vi "S4GUI_003.vi"(7 "Tab ObsEng":enum32{"Obs", "CCD modes", "Guider", "Eng"}(tab)) -> ()   [LabVIEW 2018] (continued)
              stop <- TRUE stop-if-true
              n1225 = case shown="False" w351 {
                tunnel: w350 -> [w353 w372]
                tunnel: [w354 w371] -> w347
                tunnel: w349 -> [w356 w370]
                tunnel: [w355 w369] -> w348
                frame True {
                  # "polarimetria"
                  n1226 = case shown="False" w356 {
                    selector: w356 -> [w366 w368]
                    tunnel: [w365 w368] -> w355
                    tunnel: [FALSE FALSE] -> w354
                    tunnel: w353 -> [_ _]
                    frame False {
                      w363 = 11
                      w360 = 80
                      w359 = 12900
                      # "Valor médio\ndo curso do foco."
                      n1227 = local write "Start focus"(w359) -> ()
                      n1228 = local write "Step focus"(w360) -> ()
                      n1229 = local write "#steps"(w363) -> ()
                      n1230 = Quotient & Remainder(x=w363, y=2) -> (floor(x/y)=w361:i32)  [unwired: 1 out]
                      n1231 = Multiply(x=w360, y=w361) -> (x*y=w358:i32)
                      n1232 = Add(x=w359, y=w358) -> (x+y=w357:i32)
                      n1233 = local write "Target focus 2"(w357) -> ()
                      n1234 = local write "Target focus"(w357) -> ()
                      n1235 = Not(x=w366) -> (.not. x?=w365:bool)
                    }
                    frame True {
                    }
                  }
                }
                frame False {
                  # "fotometria"
                  n1236 = case shown="False" w372 {
                    selector: w372 -> [w381 w384]
                    tunnel: [w380 w384] -> w371
                    tunnel: w370 -> [_ _]
                    tunnel: [FALSE FALSE] -> w369
                    frame False {
                      w376 = 11
                      w375 = 100
                      w374 = 13400
                      # "Valor médio\ndo curso do foco."
                      n1237 = local write "Start focus"(w374) -> ()
                      n1238 = local write "Step focus"(w375) -> ()
                      n1239 = local write "#steps"(w376) -> ()
                      n1240 = Quotient & Remainder(x=w376, y=2) -> (floor(x/y)=w378:i32)  [unwired: 1 out]
                      n1241 = Multiply(x=w375, y=w378) -> (x*y=w377:i32)
                      n1242 = Add(x=w374, y=w377) -> (x+y=w373:i32)
                      n1243 = local write "Target focus"(w373) -> ()
                      n1244 = local write "Target focus 2"(w373) -> ()
                      n1245 = Not(x=w381) -> (.not. x?=w380:bool)
                    }
                    frame True {
                    }
                  }
                }
              }
            }
            n1246 = call-dynamic "Read exit.vi"("error in (no error)"=w296, "S4GUI in"=w295) -> ("error out"=w294:errorcluster, "exit"=w293:bool, "S4GUI out"=w292:refnum<class "S4GUI.lvclass">)  [unwired: 7 in]
          }
        }
      }
      event "Lambda Selector": Mouse Down? {
        n1247 = event-data() -> ()  [unwired: 1 in, 7 out]
        n1248 = First Call?() -> (First Call?: T/F=w1992:bool)
        n1249 = case shown="True" w1992 {
          tunnel: w1994 -> [w1996 w1998]
          tunnel: [w1996 w1997] -> w1993
          frame False {
          }
          frame True {
            w2000 = u16 0 items=["OFF", "Lambda/2", "Lambda/4"] ("Lambda Selector")
            n1250 = property on="Lambda Selector" class="Ring (strict)"(error in=w1998, "Value"=w2000) -> (error out=w2001:errorcluster)  [unwired: 1 in, 1 out]
            n1251 = property on="Lambda Selector" class="Ring (strict)"(error in=w2001, "RingText.Text"="OFF" ("Boolean Text.Text")) -> (error out=w1997:errorcluster)  [unwired: 1 in, 1 out]
          }
        }
        n1252 = event-data() -> ()  [unwired: 2 in, 1 out]
      }
      event "object suffix": Key Down; "object suffix": Key Repeat {
        n1253 = event-data() -> ("Char"=w2002:i16)  [unwired: 1 in]
        "charKeyboardInteger" <- w2002
        n1254 = call-dynamic "Write charSuffix.vi"("error in (no error)"=w2005, "charSuffix"=w2002, "S4GUI in"=w2006) -> ("error out"=w2003:errorcluster, "S4GUI out"=w2004:refnum<class "S4GUI.lvclass">)  [unwired: 7 in]
      }
      event "dflat suffix": Key Down; "dflat suffix": Key Repeat {
        n1255 = event-data() -> ("Char"=w2009:i16)  [unwired: 1 in]
        n1256 = call-dynamic "Write charSuffix.vi"("error in (no error)"=w2010, "charSuffix"=w2009, "S4GUI in"=w2011) -> ("error out"=w2007:errorcluster, "S4GUI out"=w2008:refnum<class "S4GUI.lvclass">)  [unwired: 7 in]
      }
      event "sflat suffix": Key Down; "sflat suffix": Key Repeat {
        n1257 = event-data() -> ("Char"=w2014:i16)  [unwired: 1 in]
        n1258 = call-dynamic "Write charSuffix.vi"("error in (no error)"=w2015, "charSuffix"=w2014, "S4GUI in"=w2016) -> ("error out"=w2012:errorcluster, "S4GUI out"=w2013:refnum<class "S4GUI.lvclass">)  [unwired: 7 in]
      }
      event "dark suffix": Key Down; "dark suffix": Key Repeat {
        n1259 = event-data() -> ("Char"=w2019:i16)  [unwired: 1 in]
        n1260 = call-dynamic "Write charSuffix.vi"("error in (no error)"=w2020, "charSuffix"=w2019, "S4GUI in"=w2021) -> ("error out"=w2017:errorcluster, "S4GUI out"=w2018:refnum<class "S4GUI.lvclass">)  [unwired: 7 in]
      }
      event "zero suffix": Key Down; "zero suffix": Key Repeat {
        n1261 = event-data() -> ("Char"=w2024:i16)  [unwired: 1 in]
        n1262 = call-dynamic "Write charSuffix.vi"("error in (no error)"=w2025, "charSuffix"=w2024, "S4GUI in"=w2026) -> ("error out"=w2022:errorcluster, "S4GUI out"=w2023:refnum<class "S4GUI.lvclass">)  [unwired: 7 in]
      }
      event "focus suffix": Key Down; "focus suffix": Key Repeat {
        n1263 = event-data() -> ("Char"=w2029:i16)  [unwired: 1 in]
        n1264 = call-dynamic "Write charSuffix.vi"("error in (no error)"=w2030, "charSuffix"=w2029, "S4GUI in"=w2031) -> ("error out"=w2027:errorcluster, "S4GUI out"=w2028:refnum<class "S4GUI.lvclass">)  [unwired: 7 in]
      }
      event "Set CCD mode": Value Change {
        w2094 = i16 1 items=["Cooler OFF", "Cooler ON"] ("Cooler ON/OFF")
        w2108 = i16 1 items=["Cooler OFF", "Cooler ON"] ("Cooler ON/OFF")
        w2124 = i16 1 items=["Cooler OFF", "Cooler ON"] ("Cooler ON/OFF")
        w2144 = i16 1 items=["Cooler OFF", "Cooler ON"] ("Cooler ON/OFF")
        # "Sinaliza que houve requisição de SET CCD mode"
        n1265 = event-data() -> ()  [unwired: 1 in, 6 out]
        n1266 = call-dynamic "Write User Event.vi"("error in (no error)"=w2302, "User Event"="SET CCD mode ", "S4GUI in"=w2301) -> ("error out"=w2089:errorcluster, "S4GUI out"=w2088:refnum<class "S4GUI.lvclass">)  [unwired: 7 in]
        n1267 = call-dynamic "Write SET request.vi"("error in (no error)"=w2089, "SET request"=TRUE, "S4GUI in"=w2088) -> ("error out"=w2086:errorcluster, "S4GUI out"=w2087:refnum<class "S4GUI.lvclass">)  [unwired: 7 in]
        n1268 = call-dynamic "Read CCD mode.vi"("error in (no error)"=w2086, "S4GUI in"=w2087) -> ("error out"=w2299:errorcluster, "CCD mode"=w2300:T30, "S4GUI out"=w2298:refnum<class "S4GUI.lvclass">)  [unwired: 7 in]
        n1269 = Bundle By Name(cluster=w2300, "FTM"="Frame Transfer", "AQM"="AQM", "SZM"="SZM", "EM gain"="EM Gain") -> (w2297:T30)
        n1270 = call-dynamic "Write CCD mode.vi"("error in (no error)"=w2299, "CCD mode"=w2297, "S4GUI in"=w2298) -> ("error out"=w2155:errorcluster, "S4GUI out"=w2156:refnum<class "S4GUI.lvclass">)  [unwired: 7 in]
        n1271 = call-dynamic "LoadCCDmode.vi"("error in (no error)"=w2155, "S4GUI in"=w2156) -> ("error out"=w2154:errorcluster, "S4GUI out"=w2153:refnum<class "S4GUI.lvclass">)  [unwired: 8 in]
        n1272 = call-dynamic "Read Parameters CCD modes.vi"("error in (no error)"=w2154, "S4GUI in"=w2153) -> ("error out"=w2152:errorcluster, "Parameters CCD modes"=w2157:T5, "S4GUI out"=w2151:refnum<class "S4GUI.lvclass">)  [unwired: 7 in]
        n1273 = Unbundle By Name(w2157) -> ("CCD \nEM Mode"=w2289:u8, "Readout\nRate"=w2149:u8)
        n1274 = case shown="0, Default" w2289 {
          tunnel: [string[] ["30 MHz", "20 MHz", "10 MHz", "1 MHz"] ("Strings []") string[] ["1 MHz", "0.1 MHz"] ("Strings []")] -> w2290
          frame 0, Default {
          }
          frame 1 {
          }
        }
        n1275 = flat-sequence {
          tunnel: w2290 -> [w2436]
          tunnel: w2289 -> [w2437]
          tunnel: [w2437] -> w2291
          tunnel: w2157 -> [w2443]
          tunnel: [w2442] -> w2150
          tunnel: w2291 -> [w2440]
          tunnel: w2158 -> [w2441]
          tunnel: w2149 -> [w2438]
          frame #0 {
            n1276 = property on="Readout\nRate" class="Ring (strict)"("Strings []"=w2436) -> ()  [unwired: 2 in, 2 out]
            n1277 = property on="Readout\nRate" class="Ring (strict)"("Strings []"=w2436) -> ()  [unwired: 2 in, 2 out]
            n1278 = property on="Readout Rate 2" class="Ring (strict)"("Strings []"=w2436) -> ()  [unwired: 2 in, 2 out]
            n1279 = property on="Readout Rate" class="Ring (strict)"("Strings []"=w2436) -> ()  [unwired: 2 in, 2 out]
            n1280 = property on="Readout Rate 3" class="Ring (strict)"("Strings []"=w2436) -> ()  [unwired: 2 in, 2 out]
            n1281 = property on="Readout Rate 4" class="Ring (strict)"("Strings []"=w2436) -> ()  [unwired: 2 in, 2 out]
          }
          frame #1 {
            n1282 = Bundle By Name(cluster=w2443, "Readout\nRate"=w2438, "CCD \nEM Mode"=w2440) -> (w2442:T5)
            n1283 = disable-structure shown="Enabled" {
              disable-tunnel: w2441 -> [w2447 w2448]
              disable-tunnel: w2440 -> [w2446 _]
              disable-tunnel: [w2445 w2448] -> w2439
              disable-tunnel: w2438 -> [w2444 _]
              frame Disabled {
                n1284 = Bundle By Name(cluster=w2447, "Parameters.Readout\nRate"=w2444, "Parameters.CCD \nEM Mode"=w2446) -> (w2445:T8)
              }
              frame Enabled {
              }
            }
            n1285 = local write "Input Cluster"(w2439) -> ()
          }
        }
        n1286 = call-dynamic "Read InfoCCDmode.vi"("error in (no error)"=w2152, "S4GUI in"=w2151) -> ("error out"=w2292:errorcluster, "InfoCCDmode"=w2084:T2, "S4GUI out"=w2293:refnum<class "S4GUI.lvclass">)  [unwired: 7 in]
        "InfoCCDmode" <- w2084
        n1287 = Unbundle By Name(w2084) -> ("MinExpTime"=w2032:dbl)
        n1288 = call-dynamic "Read Parameters CCD modes.vi"("error in (no error)"=w2292, "S4GUI in"=w2293) -> ("error out"=w2286:errorcluster, "Parameters CCD modes"=→"Parameters CCD modes":T5, "S4GUI out"=w2287:refnum<class "S4GUI.lvclass">)  [unwired: 7 in]
        n1289 = local read "Input Cluster"() -> (w2158:T8)
        n1290 = call-dynamic "Write Parameters CCD modes.vi"("error in (no error)"=w2286, "Parameters CCD modes"=w2150, "S4GUI in"=w2287) -> ("error out"=w2265:errorcluster, "S4GUI out"=w2239:refnum<class "S4GUI.lvclass">)  [unwired: 7 in]
        n1291 = Unbundle By Name(w2150) -> ("Frame\nTransfer"=w2193:bool, "Pre-amplification\nGain"=w2192:u8, "Readout\nRate"=w2191:u8, "CCD \nEM Mode"=w2190:u8, "CCD\nEM Gain"=w2189:u16, "Image \nInitial Line"=w2188:u16, "Image\nInitial Column"=w2187:u16, "Image\nFinal Line"=w2176:u16, "Image\nFInal Column"=w2186:u16, "Vertical\nBinning"=w2185:u16, "Horizontal\nBinning"=w2184:u16)
        n1292 = call-dynamic "Read AcquisitionA.vi"("error in (no error)"=w2265, "S4ACS_GUI in"=w2239) -> ("error out"=w2174:errorcluster, "Acquisition.lvclass"=w2175:refnum<class "Acquisition.lvclass">, "S4ACS_GUI out"=w2285:refnum<class "S4GUI.lvclass">)  [unwired: 7 in]
        n1293 = call-dynamic "Read enabled.vi"("error in (no error)"=w2174, "Server in"=w2175) -> ("error out"=w2173:errorcluster, "enabled"=w2171:bool, "Server out"=w2172:refnum<class "Acquisition.lvclass">)  [unwired: 7 in]
        n1294 = call-dynamic "Read Channel.vi"("error in (no error)"=w2173, "Acquisition in"=w2172) -> ("error out"=w2282:errorcluster, "Channel.lvclass"=w2283:refnum<class "Channel.lvclass">, "Acquisition out"=w2284:refnum<class "Acquisition.lvclass">)  [unwired: 7 in]
        n1295 = call-dynamic "Read Interface.vi"("error in (no error)"=w2282, "Channel in"=w2283) -> ("error out"=w2268:errorcluster, "Interface.lvclass"=w2269:refnum<class "Interface.lvclass">, "Channel out"=w2263:refnum<class "Channel.lvclass">)  [unwired: 7 in]
        n1296 = call-dynamic "Write PREV_FT.vi"("error in (no error)"=w2268, "PREV_FT"=w2193, "Interface in"=w2269) -> ("error out"=w2147:errorcluster, "Interface out"=w2146:refnum<class "Interface.lvclass">)  [unwired: 7 in]
        n1297 = call-dynamic "Write Cooler ON_OFF.vi"("error in (no error)"=w2147, "Cooler ON/OFF"=w2144, "Interface in"=w2146) -> ("error out"=w2145:errorcluster, "Interface out"=w2143:refnum<class "Interface.lvclass">)  [unwired: 7 in]
        n1298 = call-dynamic "Read target cluster.vi"("error in (no error)"=w2145, "Channel in"=w2263) -> ("error out"=w2261:errorcluster, "target cluster"=w2260:T31, "Channel out"=w2262:refnum<class "Channel.lvclass">)  [unwired: 7 in]
        n1299 = Bundle By Name(cluster=w2260, "FRAME_TRANSFER"=w2193, "PREAMP"=w2192, "READOUT_RATE"=w2191, "EM_MODE"=w2190, "EM_GAIN"=w2189, "INITIAL_LINE"=w2188, "INITIAL_COLUMN"=w2187, "FINAL_LINE"=w2176, "FINAL_COLUMN"=w2186, "VBIN"=w2185, "HBIN"=w2184) -> (w2140:T31)
        n1300 = call-dynamic "Write target cluster.vi"("error in (no error)"=w2261, "target cluster"=w2140, "Channel in"=w2262) -> ("error out"=w2141:errorcluster, "Channel out"=w2267:refnum<class "Channel.lvclass">)  [unwired: 7 in]
        n1301 = call-dynamic "Set CCD_Config.vi"("error in (no error)"=w2141, "input cluster"=w2140, "Interface in"=w2143) -> ("error out"=w2130:errorcluster, "Interface out"=w2142:refnum<class "Interface.lvclass">)  [unwired: 7 in]
        n1302 = Flatten To String(anything=w2140, error in (no error)=w2141) -> (data string=w2277:string)  [unwired: 2 in, 2 out]
        n1303 = call "Write flatted cluster.vi"("error in (no error)"=w2130, "flatted cluster"=w2277, "Interface in"=w2142) -> ("error out"=w2079:errorcluster, "Interface out"=w2080:refnum<class "Interface.lvclass">)  [unwired: 7 in]
        n1304 = call "Read Exposure Time.vi"("error in (no error)"=w2079, "Interface in"=w2080) -> ("error out"=w2077:errorcluster, "Exposure Time"=w2082:dbl, "Interface out"=w2078:refnum<class "Interface.lvclass">)  [unwired: 7 in]
        n1305 = Greater Or Equal?(x=w2082, y=w2032) -> (x >= y?=w2083:bool)
        n1306 = Select(t=w2082, s=w2083, f=w2032) -> (s? t:f=w2081:dbl)
        n1307 = local write "Exptime ch1"(w2081) -> ()
        n1308 = call "Write Exposure Time.vi"("error in (no error)"=w2077, "Exposure Time"=w2081, "Interface in"=w2078) -> ("error out"=w2076:errorcluster, "Interface out"=w2075:refnum<class "Interface.lvclass">)  [unwired: 7 in]
        n1309 = call-dynamic "Write Interface.vi"("error in (no error)"=w2076, "Interface.lvclass"=w2075, "Channel in"=w2267) -> ("error out"=w2273:errorcluster, "Channel out"=w2275:refnum<class "Channel.lvclass">)  [unwired: 7 in]
        n1310 = call "Write section_name.vi"("error in (no error)"=w2273, "section_name"="CCD_ACS1", "Channel in"=w2275) -> ("error out"=w2272:errorcluster, "Channel out"=w2274:refnum<class "Channel.lvclass">)  [unwired: 7 in]
        n1311 = call-dynamic "save config.vi"("error in (no error)"=w2272, "file config"="lastsaved.cfg", "Channel in"=w2274) -> ("error out"=w2138:errorcluster, "Channel out"=w2139:refnum<class "Channel.lvclass">)  [unwired: 7 in]
        n1312 = call-dynamic "ValidateConfig.vi"("error in (no error)"=w2138, "Channel in"=w2139) -> ("error out"=w2136:errorcluster, "Channel out"=w2137:refnum<class "Channel.lvclass">)  [unwired: 7 in, 1 out]
        n1313 = call-dynamic "Save Temp.vi"("error in (no error)"=w2136, "temp file"="lasttemp.cfg" ("file config"), "Channel in"=w2137) -> ("error out"=w2135:errorcluster, "Channel out"=w2134:refnum<class "Channel.lvclass">)  [unwired: 7 in]
        n1314 = case shown="True" w2171 {
          tunnel: [w2404 w2429] -> w2281
          tunnel: [w2403 w2428] -> w2280
          tunnel: w2134 -> [w2404 w2427]
          tunnel: w2135 -> [w2403 w2426]
          frame False {
          }
          frame True {
            # "Esvazia\na fila."
            n1315 = call-dynamic "Read State Machine.vi"("error in (no error)"=w2426, "Device in"=w2427) -> ("error out"=w2420:errorcluster, "State Machine.lvclass"=w2423:refnum<class "State Machine.lvclass">, "Device out"=w2433:refnum<class "Channel.lvclass">)  [unwired: 7 in]
            n1316 = call-dynamic "Read ref StatesQueue.vi"("error in (no error)"=w2420, "State Machine in"=w2423) -> ("error out"=w2411:errorcluster, "ref StatesQueue"=w2413:refnum<queue>, "State Machine out"=w2422:refnum<class "State Machine.lvclass">)  [unwired: 7 in]
            n1317 = Flush Queue(queue=w2413, error in (no error)=w2411) -> (queue out=w2412:refnum<queue>, error out=w2410:errorcluster)  [unwired: 1 out]
            n1318 = Enqueue Element(queue=w2412, element=u32 60 ("State"), error in (no error)=w2410) -> (queue out=w2425:refnum<queue>, error out=w2419:errorcluster)  [unwired: 1 in, 1 out]
            n1319 = Enqueue Element(queue=w2425, element=u32 45 ("State"), error in (no error)=w2419) -> (queue out=w2424:refnum<queue>, error out=w2418:errorcluster)  [unwired: 1 in, 1 out]
            n1320 = Enqueue Element(queue=w2424, element=u32 35 ("State"), error in (no error)=w2418) -> (queue out=w2408:refnum<queue>, error out=w2407:errorcluster)  [unwired: 1 in, 1 out]
            n1321 = Enqueue Element(queue=w2408, element=u32 37 ("State"), error in (no error)=w2407) -> (queue out=w2405:refnum<queue>, error out=w2406:errorcluster)  [unwired: 1 in, 1 out]
            n1322 = call-dynamic "Write ref StatesQueue.vi"("error in (no error)"=w2406, "ref StatesQueue"=w2405, "State Machine in"=w2422) -> ("error out"=w2414:errorcluster, "State Machine out"=w2421:refnum<class "State Machine.lvclass">)  [unwired: 7 in]
            n1323 = disable-structure shown="Enabled" {
              disable-tunnel: [0 ("State") 45] -> w2430
              frame Enabled {
                # "Vai pra 0 para que\nos estados da fila \nsejam retirados."
              }
              frame Disabled {
                # "Verifica Texp\nantes de tudo."
              }
            }
            n1324 = call-dynamic "Write State.vi"("error in (no error)"=w2414, "State"=w2430, "State Machine in"=w2421) -> ("error out"=w2431:errorcluster, "State Machine out"=w2432:refnum<class "State Machine.lvclass">)  [unwired: 7 in]
            n1325 = call-dynamic "Write State Machine.vi"("error in (no error)"=w2431, "State Machine.lvclass"=w2432, "Device in"=w2433) -> ("error out"=w2428:errorcluster, "Device out"=w2429:refnum<class "Channel.lvclass">)  [unwired: 7 in]
          }
        }
        n1326 = call-dynamic "Write Channel.vi"("error in (no error)"=w2280, "Channel.lvclass"=w2281, "Acquisition in"=w2284) -> ("error out"=w2279:errorcluster, "Acquisition out"=w2278:refnum<class "Acquisition.lvclass">)  [unwired: 7 in]
        n1327 = call-dynamic "Write AcquisitionA.vi"("error in (no error)"=w2279, "Acquisition.lvclass"=w2278, "S4ACS_GUI in"=w2285) -> ("error out"=w2181:errorcluster, "S4ACS_GUI out"=w2238:refnum<class "S4GUI.lvclass">)  [unwired: 7 in]
        n1328 = call "Read AcquisitionB.vi"("error in (no error)"=errorcluster {"status"=FALSE, "code"=0, "source"=""}, "S4ACS_GUI in"=w2238) -> ("error out"=w2167:errorcluster, "Acquisition.lvclass"=w2170:refnum<class "Acquisition.lvclass">, "S4ACS_GUI out"=w2259:refnum<class "S4GUI.lvclass">)  [unwired: 7 in]
        n1329 = call-dynamic "Read enabled.vi"("error in (no error)"=w2167, "Server in"=w2170) -> ("error out"=w2168:errorcluster, "enabled"=w2060:bool, "Server out"=w2169:refnum<class "Acquisition.lvclass">)  [unwired: 7 in]
        n1330 = call-dynamic "Read Channel.vi"("error in (no error)"=w2168, "Acquisition in"=w2169) -> ("error out"=w2256:errorcluster, "Channel.lvclass"=w2257:refnum<class "Channel.lvclass">, "Acquisition out"=w2258:refnum<class "Acquisition.lvclass">)  [unwired: 7 in]
        n1331 = call-dynamic "Read Interface.vi"("error in (no error)"=w2256, "Channel in"=w2257) -> ("error out"=w2245:errorcluster, "Interface.lvclass"=w2246:refnum<class "Interface.lvclass">, "Channel out"=w2243:refnum<class "Channel.lvclass">)  [unwired: 7 in]
        n1332 = call-dynamic "Write PREV_FT.vi"("error in (no error)"=w2245, "PREV_FT"=w2193, "Interface in"=w2246) -> ("error out"=w2125:errorcluster, "Interface out"=w2127:refnum<class "Interface.lvclass">)  [unwired: 7 in]
        n1333 = call-dynamic "Write Cooler ON_OFF.vi"("error in (no error)"=w2125, "Cooler ON/OFF"=w2124, "Interface in"=w2127) -> ("error out"=w2123:errorcluster, "Interface out"=w2126:refnum<class "Interface.lvclass">)  [unwired: 7 in]
        n1334 = call-dynamic "Read target cluster.vi"("error in (no error)"=w2123, "Channel in"=w2243) -> ("error out"=w2241:errorcluster, "target cluster"=w2240:T31, "Channel out"=w2242:refnum<class "Channel.lvclass">)  [unwired: 7 in]
        n1335 = Bundle By Name(cluster=w2240, "FRAME_TRANSFER"=w2193, "PREAMP"=w2192, "READOUT_RATE"=w2191, "EM_MODE"=w2190, "EM_GAIN"=w2189, "INITIAL_LINE"=w2188, "INITIAL_COLUMN"=w2187, "FINAL_LINE"=w2176, "FINAL_COLUMN"=w2186, "VBIN"=w2185, "HBIN"=w2184) -> (w2128:T31)
        n1336 = call-dynamic "Write target cluster.vi"("error in (no error)"=w2241, "target cluster"=w2128, "Channel in"=w2242) -> ("error out"=w2131:errorcluster, "Channel out"=w2244:refnum<class "Channel.lvclass">)  [unwired: 7 in]
        n1337 = call-dynamic "Set CCD_Config.vi"("error in (no error)"=w2131, "input cluster"=w2128, "Interface in"=w2126) -> ("error out"=w2129:errorcluster, "Interface out"=w2132:refnum<class "Interface.lvclass">)  [unwired: 7 in]
        n1338 = Flatten To String(anything=w2128, error in (no error)=w2131) -> (data string=w2253:string)  [unwired: 2 in, 2 out]
        n1339 = call "Write flatted cluster.vi"("error in (no error)"=w2129, "flatted cluster"=w2253, "Interface in"=w2132) -> ("error out"=w2053:errorcluster, "Interface out"=w2054:refnum<class "Interface.lvclass">)  [unwired: 7 in]
        n1340 = call "Read Exposure Time.vi"("error in (no error)"=w2053, "Interface in"=w2054) -> ("error out"=w2074:errorcluster, "Exposure Time"=w2055:dbl, "Interface out"=w2073:refnum<class "Interface.lvclass">)  [unwired: 7 in]
        n1341 = Greater Or Equal?(x=w2055, y=w2032) -> (x >= y?=w2071:bool)
        n1342 = Select(t=w2055, s=w2071, f=w2032) -> (s? t:f=w2072:dbl)
        n1343 = local write "Exptime ch2"(w2072) -> ()
        n1344 = call "Write Exposure Time.vi"("error in (no error)"=w2074, "Exposure Time"=w2072, "Interface in"=w2073) -> ("error out"=w2052:errorcluster, "Interface out"=w2051:refnum<class "Interface.lvclass">)  [unwired: 7 in]
        n1345 = call-dynamic "Write Interface.vi"("error in (no error)"=w2052, "Interface.lvclass"=w2051, "Channel in"=w2244) -> ("error out"=w2249:errorcluster, "Channel out"=w2251:refnum<class "Channel.lvclass">)  [unwired: 7 in]
        n1346 = call "Write section_name.vi"("error in (no error)"=w2249, "section_name"="CCD_ACS2", "Channel in"=w2251) -> ("error out"=w2248:errorcluster, "Channel out"=w2250:refnum<class "Channel.lvclass">)  [unwired: 7 in]
        n1347 = call-dynamic "save config.vi"("error in (no error)"=w2248, "file config"="lastsaved.cfg", "Channel in"=w2250) -> ("error out"=w2118:errorcluster, "Channel out"=w2119:refnum<class "Channel.lvclass">)  [unwired: 7 in]
        n1348 = call-dynamic "ValidateConfig.vi"("error in (no error)"=w2118, "Channel in"=w2119) -> ("error out"=w2121:errorcluster, "Channel out"=w2122:refnum<class "Channel.lvclass">)  [unwired: 7 in, 1 out]
        n1349 = call-dynamic "Save Temp.vi"("error in (no error)"=w2121, "temp file"="lasttemp.cfg" ("file config"), "Channel in"=w2122) -> ("error out"=w2058:errorcluster, "Channel out"=w2059:refnum<class "Channel.lvclass">)  [unwired: 7 in]
        n1350 = case shown="True" w2060 {
          tunnel: [w2338 w2363] -> w2057
          tunnel: [w2337 w2362] -> w2056
          tunnel: w2059 -> [w2338 w2361]
          tunnel: w2058 -> [w2337 w2360]
          frame False {
          }
          frame True {
            # "Esvazia\na fila."
            n1351 = call-dynamic "Read State Machine.vi"("error in (no error)"=w2360, "Device in"=w2361) -> ("error out"=w2354:errorcluster, "State Machine.lvclass"=w2357:refnum<class "State Machine.lvclass">, "Device out"=w2367:refnum<class "Channel.lvclass">)  [unwired: 7 in]
            n1352 = call-dynamic "Read ref StatesQueue.vi"("error in (no error)"=w2354, "State Machine in"=w2357) -> ("error out"=w2344:errorcluster, "ref StatesQueue"=w2346:refnum<queue>, "State Machine out"=w2356:refnum<class "State Machine.lvclass">)  [unwired: 7 in]
            n1353 = Flush Queue(queue=w2346, error in (no error)=w2344) -> (queue out=w2345:refnum<queue>, error out=w2343:errorcluster)  [unwired: 1 out]
            n1354 = Enqueue Element(queue=w2345, element=u32 60 ("State"), error in (no error)=w2343) -> (queue out=w2359:refnum<queue>, error out=w2353:errorcluster)  [unwired: 1 in, 1 out]
            n1355 = Enqueue Element(queue=w2359, element=u32 45 ("State"), error in (no error)=w2353) -> (queue out=w2358:refnum<queue>, error out=w2352:errorcluster)  [unwired: 1 in, 1 out]
            n1356 = Enqueue Element(queue=w2358, element=u32 35 ("State"), error in (no error)=w2352) -> (queue out=w2351:refnum<queue>, error out=w2341:errorcluster)  [unwired: 1 in, 1 out]
            n1357 = Enqueue Element(queue=w2351, element=u32 37, error in (no error)=w2341) -> (queue out=w2342:refnum<queue>, error out=w2340:errorcluster)  [unwired: 1 in, 1 out]
            n1358 = call-dynamic "Write ref StatesQueue.vi"("error in (no error)"=w2340, "ref StatesQueue"=w2342, "State Machine in"=w2356) -> ("error out"=w2347:errorcluster, "State Machine out"=w2355:refnum<class "State Machine.lvclass">)  [unwired: 7 in]
            n1359 = disable-structure shown="Enabled" {
              disable-tunnel: [0 ("State") 45] -> w2364
              frame Enabled {
                # "Vai pra 0 para que\nos estados da fila \nsejam retirados."
              }
              frame Disabled {
                # "Verifica Texp\nantes de tudo."
              }
            }
            n1360 = call-dynamic "Write State.vi"("error in (no error)"=w2347, "State"=w2364, "State Machine in"=w2355) -> ("error out"=w2365:errorcluster, "State Machine out"=w2366:refnum<class "State Machine.lvclass">)  [unwired: 7 in]
            n1361 = call-dynamic "Write State Machine.vi"("error in (no error)"=w2365, "State Machine.lvclass"=w2366, "Device in"=w2367) -> ("error out"=w2362:errorcluster, "Device out"=w2363:refnum<class "Channel.lvclass">)  [unwired: 7 in]
          }
        }
        n1362 = call-dynamic "Write Channel.vi"("error in (no error)"=w2056, "Channel.lvclass"=w2057, "Acquisition in"=w2258) -> ("error out"=w2255:errorcluster, "Acquisition out"=w2254:refnum<class "Acquisition.lvclass">)  [unwired: 7 in]
        n1363 = call "Write AcquisitionB.vi"("error in (no error)"=w2255, "Acquisition.lvclass"=w2254, "S4ACS_GUI in"=w2259) -> ("error out"=w2180:errorcluster, "S4ACS_GUI out"=w2215:refnum<class "S4GUI.lvclass">)  [unwired: 7 in]
        n1364 = call-dynamic "Read AcquisitionC.vi"("error in (no error)"=errorcluster {"status"=FALSE, "code"=0, "source"=""}, "S4ACS_GUI in"=w2215) -> ("error out"=w2164:errorcluster, "Acquisition.lvclass"=w2166:refnum<class "Acquisition.lvclass">, "S4ACS_GUI out"=w2236:refnum<class "S4GUI.lvclass">)  [unwired: 7 in]
        n1365 = call-dynamic "Read enabled.vi"("error in (no error)"=w2164, "Server in"=w2166) -> ("error out"=w2163:errorcluster, "enabled"=w2050:bool, "Server out"=w2165:refnum<class "Acquisition.lvclass">)  [unwired: 7 in]
        n1366 = call-dynamic "Read Channel.vi"("error in (no error)"=w2163, "Acquisition in"=w2165) -> ("error out"=w2233:errorcluster, "Channel.lvclass"=w2234:refnum<class "Channel.lvclass">, "Acquisition out"=w2235:refnum<class "Acquisition.lvclass">)  [unwired: 7 in]
        n1367 = call-dynamic "Read Interface.vi"("error in (no error)"=w2233, "Channel in"=w2234) -> ("error out"=w2222:errorcluster, "Interface.lvclass"=w2223:refnum<class "Interface.lvclass">, "Channel out"=w2220:refnum<class "Channel.lvclass">)  [unwired: 7 in]
        n1368 = call-dynamic "Write PREV_FT.vi"("error in (no error)"=w2222, "PREV_FT"=w2193, "Interface in"=w2223) -> ("error out"=w2105:errorcluster, "Interface out"=w2107:refnum<class "Interface.lvclass">)  [unwired: 7 in]
        n1369 = call-dynamic "Write Cooler ON_OFF.vi"("error in (no error)"=w2105, "Cooler ON/OFF"=w2108, "Interface in"=w2107) -> ("error out"=w2104:errorcluster, "Interface out"=w2106:refnum<class "Interface.lvclass">)  [unwired: 7 in]
        n1370 = call-dynamic "Read target cluster.vi"("error in (no error)"=w2104, "Channel in"=w2220) -> ("error out"=w2218:errorcluster, "target cluster"=w2217:T31, "Channel out"=w2219:refnum<class "Channel.lvclass">)  [unwired: 7 in]
        n1371 = Bundle By Name(cluster=w2217, "FRAME_TRANSFER"=w2193, "PREAMP"=w2192, "READOUT_RATE"=w2191, "EM_MODE"=w2190, "EM_GAIN"=w2189, "INITIAL_LINE"=w2188, "INITIAL_COLUMN"=w2187, "FINAL_LINE"=w2176, "FINAL_COLUMN"=w2186, "VBIN"=w2185, "HBIN"=w2184) -> (w2112:T31)
        n1372 = call-dynamic "Write target cluster.vi"("error in (no error)"=w2218, "target cluster"=w2112, "Channel in"=w2219) -> ("error out"=w2111:errorcluster, "Channel out"=w2221:refnum<class "Channel.lvclass">)  [unwired: 7 in]
        n1373 = call-dynamic "Set CCD_Config.vi"("error in (no error)"=w2111, "input cluster"=w2112, "Interface in"=w2106) -> ("error out"=w2110:errorcluster, "Interface out"=w2109:refnum<class "Interface.lvclass">)  [unwired: 7 in]
        n1374 = Flatten To String(anything=w2112, error in (no error)=w2111) -> (data string=w2230:string)  [unwired: 2 in, 2 out]
        n1375 = call "Write flatted cluster.vi"("error in (no error)"=w2110, "flatted cluster"=w2230, "Interface in"=w2109) -> ("error out"=w2044:errorcluster, "Interface out"=w2045:refnum<class "Interface.lvclass">)  [unwired: 7 in]
        n1376 = call "Read Exposure Time.vi"("error in (no error)"=w2044, "Interface in"=w2045) -> ("error out"=w2066:errorcluster, "Exposure Time"=w2069:dbl, "Interface out"=w2067:refnum<class "Interface.lvclass">)  [unwired: 7 in]
        n1377 = Greater Or Equal?(x=w2069, y=w2032) -> (x >= y?=w2070:bool)
        n1378 = Select(t=w2069, s=w2070, f=w2032) -> (s? t:f=w2068:dbl)
        n1379 = local write "Exptime ch3"(w2068) -> ()
        n1380 = call "Write Exposure Time.vi"("error in (no error)"=w2066, "Exposure Time"=w2068, "Interface in"=w2067) -> ("error out"=w2042:errorcluster, "Interface out"=w2043:refnum<class "Interface.lvclass">)  [unwired: 7 in]
        n1381 = call-dynamic "Write Interface.vi"("error in (no error)"=w2042, "Interface.lvclass"=w2043, "Channel in"=w2221) -> ("error out"=w2226:errorcluster, "Channel out"=w2228:refnum<class "Channel.lvclass">)  [unwired: 7 in]
        n1382 = call "Write section_name.vi"("error in (no error)"=w2226, "section_name"="CCD_ACS3", "Channel in"=w2228) -> ("error out"=w2225:errorcluster, "Channel out"=w2227:refnum<class "Channel.lvclass">)  [unwired: 7 in]
        n1383 = call-dynamic "save config.vi"("error in (no error)"=w2225, "file config"="lastsaved.cfg", "Channel in"=w2227) -> ("error out"=w2113:errorcluster, "Channel out"=w2114:refnum<class "Channel.lvclass">)  [unwired: 7 in]
        n1384 = call-dynamic "ValidateConfig.vi"("error in (no error)"=w2113, "Channel in"=w2114) -> ("error out"=w2116:errorcluster, "Channel out"=w2117:refnum<class "Channel.lvclass">)  [unwired: 7 in, 1 out]
        n1385 = call-dynamic "Save Temp.vi"("error in (no error)"=w2116, "temp file"="lasttemp.cfg" ("file config"), "Channel in"=w2117) -> ("error out"=w2048:errorcluster, "Channel out"=w2049:refnum<class "Channel.lvclass">)  [unwired: 7 in]
        n1386 = case shown="True" w2050 {
          tunnel: [w2305 w2330] -> w2047
          tunnel: [w2304 w2329] -> w2046
          tunnel: w2049 -> [w2305 w2328]
          tunnel: w2048 -> [w2304 w2327]
          frame False {
          }
          frame True {
            # "Esvazia\na fila."
            n1387 = call-dynamic "Read State Machine.vi"("error in (no error)"=w2327, "Device in"=w2328) -> ("error out"=w2321:errorcluster, "State Machine.lvclass"=w2324:refnum<class "State Machine.lvclass">, "Device out"=w2334:refnum<class "Channel.lvclass">)  [unwired: 7 in]
            n1388 = call-dynamic "Read ref StatesQueue.vi"("error in (no error)"=w2321, "State Machine in"=w2324) -> ("error out"=w2311:errorcluster, "ref StatesQueue"=w2313:refnum<queue>, "State Machine out"=w2323:refnum<class "State Machine.lvclass">)  [unwired: 7 in]
            n1389 = Flush Queue(queue=w2313, error in (no error)=w2311) -> (queue out=w2312:refnum<queue>, error out=w2310:errorcluster)  [unwired: 1 out]
            n1390 = Enqueue Element(queue=w2312, element=u32 60 ("State"), error in (no error)=w2310) -> (queue out=w2326:refnum<queue>, error out=w2320:errorcluster)  [unwired: 1 in, 1 out]
            n1391 = Enqueue Element(queue=w2326, element=u32 45 ("State"), error in (no error)=w2320) -> (queue out=w2325:refnum<queue>, error out=w2319:errorcluster)  [unwired: 1 in, 1 out]
            n1392 = Enqueue Element(queue=w2325, element=u32 35 ("State"), error in (no error)=w2319) -> (queue out=w2318:refnum<queue>, error out=w2308:errorcluster)  [unwired: 1 in, 1 out]
            n1393 = Enqueue Element(queue=w2318, element=u32 37, error in (no error)=w2308) -> (queue out=w2309:refnum<queue>, error out=w2307:errorcluster)  [unwired: 1 in, 1 out]
            n1394 = call-dynamic "Write ref StatesQueue.vi"("error in (no error)"=w2307, "ref StatesQueue"=w2309, "State Machine in"=w2323) -> ("error out"=w2314:errorcluster, "State Machine out"=w2322:refnum<class "State Machine.lvclass">)  [unwired: 7 in]
            n1395 = disable-structure shown="Enabled" {
              disable-tunnel: [0 ("State") 45] -> w2331
              frame Enabled {
                # "Vai pra 0 para que\nos estados da fila \nsejam retirados."
              }
              frame Disabled {
                # "Verifica Texp\nantes de tudo."
              }
            }
            n1396 = call-dynamic "Write State.vi"("error in (no error)"=w2314, "State"=w2331, "State Machine in"=w2322) -> ("error out"=w2332:errorcluster, "State Machine out"=w2333:refnum<class "State Machine.lvclass">)  [unwired: 7 in]
            n1397 = call-dynamic "Write State Machine.vi"("error in (no error)"=w2332, "State Machine.lvclass"=w2333, "Device in"=w2334) -> ("error out"=w2329:errorcluster, "Device out"=w2330:refnum<class "Channel.lvclass">)  [unwired: 7 in]
          }
        }
        n1398 = call-dynamic "Write Channel.vi"("error in (no error)"=w2046, "Channel.lvclass"=w2047, "Acquisition in"=w2235) -> ("error out"=w2232:errorcluster, "Acquisition out"=w2231:refnum<class "Acquisition.lvclass">)  [unwired: 7 in]
        n1399 = call-dynamic "Write AcquisitionC.vi"("error in (no error)"=w2232, "Acquisition.lvclass"=w2231, "S4ACS_GUI in"=w2236) -> ("error out"=w2179:errorcluster, "S4ACS_GUI out"=w2183:refnum<class "S4GUI.lvclass">)  [unwired: 7 in]
        n1400 = call-dynamic "Read AcquisitionD.vi"("error in (no error)"=errorcluster {"status"=FALSE, "code"=0, "source"=""}, "S4ACS_GUI in"=w2183) -> ("error out"=w2160:errorcluster, "Acquisition.lvclass"=w2162:refnum<class "Acquisition.lvclass">, "S4ACS_GUI out"=w2214:refnum<class "S4GUI.lvclass">)  [unwired: 7 in]
        n1401 = call-dynamic "Read enabled.vi"("error in (no error)"=w2160, "Server in"=w2162) -> ("error out"=w2159:errorcluster, "enabled"=w2041:bool, "Server out"=w2161:refnum<class "Acquisition.lvclass">)  [unwired: 7 in]
        n1402 = call-dynamic "Read Channel.vi"("error in (no error)"=w2159, "Acquisition in"=w2161) -> ("error out"=w2211:errorcluster, "Channel.lvclass"=w2212:refnum<class "Channel.lvclass">, "Acquisition out"=w2213:refnum<class "Acquisition.lvclass">)  [unwired: 7 in]
        n1403 = call-dynamic "Read Interface.vi"("error in (no error)"=w2211, "Channel in"=w2212) -> ("error out"=w2200:errorcluster, "Interface.lvclass"=w2201:refnum<class "Interface.lvclass">, "Channel out"=w2198:refnum<class "Channel.lvclass">)  [unwired: 7 in]
        n1404 = call-dynamic "Write PREV_FT.vi"("error in (no error)"=w2200, "PREV_FT"=w2193, "Interface in"=w2201) -> ("error out"=w2093:errorcluster, "Interface out"=w2092:refnum<class "Interface.lvclass">)  [unwired: 7 in]
        n1405 = call-dynamic "Write Cooler ON_OFF.vi"("error in (no error)"=w2093, "Cooler ON/OFF"=w2094, "Interface in"=w2092) -> ("error out"=w2090:errorcluster, "Interface out"=w2091:refnum<class "Interface.lvclass">)  [unwired: 7 in]
        n1406 = call-dynamic "Read target cluster.vi"("error in (no error)"=w2090, "Channel in"=w2198) -> ("error out"=w2196:errorcluster, "target cluster"=w2195:T31, "Channel out"=w2197:refnum<class "Channel.lvclass">)  [unwired: 7 in]
        n1407 = Bundle By Name(cluster=w2195, "FRAME_TRANSFER"=w2193, "PREAMP"=w2192, "READOUT_RATE"=w2191, "EM_MODE"=w2190, "EM_GAIN"=w2189, "INITIAL_LINE"=w2188, "INITIAL_COLUMN"=w2187, "FINAL_LINE"=w2176, "FINAL_COLUMN"=w2186, "VBIN"=w2185, "HBIN"=w2184) -> (w2095:T31)
        n1408 = call-dynamic "Write target cluster.vi"("error in (no error)"=w2196, "target cluster"=w2095, "Channel in"=w2197) -> ("error out"=w2096:errorcluster, "Channel out"=w2199:refnum<class "Channel.lvclass">)  [unwired: 7 in]
        n1409 = call-dynamic "Set CCD_Config.vi"("error in (no error)"=w2096, "input cluster"=w2095, "Interface in"=w2091) -> ("error out"=w2097:errorcluster, "Interface out"=w2098:refnum<class "Interface.lvclass">)  [unwired: 7 in]
        n1410 = Flatten To String(anything=w2095, error in (no error)=w2096) -> (data string=w2208:string)  [unwired: 2 in, 2 out]
        n1411 = call "Write flatted cluster.vi"("error in (no error)"=w2097, "flatted cluster"=w2208, "Interface in"=w2098) -> ("error out"=w2035:errorcluster, "Interface out"=w2036:refnum<class "Interface.lvclass">)  [unwired: 7 in]
        n1412 = call "Read Exposure Time.vi"("error in (no error)"=w2035, "Interface in"=w2036) -> ("error out"=w2065:errorcluster, "Exposure Time"=w2062:dbl, "Interface out"=w2064:refnum<class "Interface.lvclass">)  [unwired: 7 in]
        n1413 = Greater Or Equal?(x=w2062, y=w2032) -> (x >= y?=w2061:bool)
        n1414 = Select(t=w2062, s=w2061, f=w2032) -> (s? t:f=w2063:dbl)
        n1415 = local write "Exptime ch4"(w2063) -> ()
        n1416 = call "Write Exposure Time.vi"("error in (no error)"=w2065, "Exposure Time"=w2063, "Interface in"=w2064) -> ("error out"=w2033:errorcluster, "Interface out"=w2034:refnum<class "Interface.lvclass">)  [unwired: 7 in]
        n1417 = call-dynamic "Write Interface.vi"("error in (no error)"=w2033, "Interface.lvclass"=w2034, "Channel in"=w2199) -> ("error out"=w2204:errorcluster, "Channel out"=w2206:refnum<class "Channel.lvclass">)  [unwired: 7 in]
        n1418 = call "Write section_name.vi"("error in (no error)"=w2204, "section_name"="CCD_ACS4", "Channel in"=w2206) -> ("error out"=w2203:errorcluster, "Channel out"=w2205:refnum<class "Channel.lvclass">)  [unwired: 7 in]
        n1419 = call-dynamic "save config.vi"("error in (no error)"=w2203, "file config"="lastsaved.cfg", "Channel in"=w2205) -> ("error out"=w2099:errorcluster, "Channel out"=w2100:refnum<class "Channel.lvclass">)  [unwired: 7 in]
        n1420 = call-dynamic "ValidateConfig.vi"("error in (no error)"=w2099, "Channel in"=w2100) -> ("error out"=w2102:errorcluster, "Channel out"=w2103:refnum<class "Channel.lvclass">)  [unwired: 7 in, 1 out]
        n1421 = call-dynamic "Save Temp.vi"("error in (no error)"=w2102, "temp file"="lasttemp.cfg" ("file config"), "Channel in"=w2103) -> ("error out"=w2038:errorcluster, "Channel out"=w2037:refnum<class "Channel.lvclass">)  [unwired: 7 in]
        n1422 = case shown="True" w2041 {
          tunnel: [w2370 w2396] -> w2040
          tunnel: [w2371 w2395] -> w2039
          tunnel: w2038 -> [w2371 w2394]
          tunnel: w2037 -> [w2370 w2376]
          frame False {
          }
          frame True {
            # "Esvazia\na fila."
            n1423 = call-dynamic "Read State Machine.vi"("error in (no error)"=w2394, "Device in"=w2376) -> ("error out"=w2388:errorcluster, "State Machine.lvclass"=w2391:refnum<class "State Machine.lvclass">, "Device out"=w2400:refnum<class "Channel.lvclass">)  [unwired: 7 in]
            n1424 = call-dynamic "Read ref StatesQueue.vi"("error in (no error)"=w2388, "State Machine in"=w2391) -> ("error out"=w2378:errorcluster, "ref StatesQueue"=w2380:refnum<queue>, "State Machine out"=w2390:refnum<class "State Machine.lvclass">)  [unwired: 7 in]
            n1425 = Flush Queue(queue=w2380, error in (no error)=w2378) -> (queue out=w2379:refnum<queue>, error out=w2377:errorcluster)  [unwired: 1 out]
            n1426 = Enqueue Element(queue=w2379, element=u32 60 ("State"), error in (no error)=w2377) -> (queue out=w2393:refnum<queue>, error out=w2387:errorcluster)  [unwired: 1 in, 1 out]
            n1427 = Enqueue Element(queue=w2393, element=u32 45 ("State"), error in (no error)=w2387) -> (queue out=w2392:refnum<queue>, error out=w2386:errorcluster)  [unwired: 1 in, 1 out]
            n1428 = Enqueue Element(queue=w2392, element=u32 35 ("State"), error in (no error)=w2386) -> (queue out=w2385:refnum<queue>, error out=w2374:errorcluster)  [unwired: 1 in, 1 out]
            n1429 = Enqueue Element(queue=w2385, element=u32 37, error in (no error)=w2374) -> (queue out=w2375:refnum<queue>, error out=w2373:errorcluster)  [unwired: 1 in, 1 out]
            n1430 = call-dynamic "Write ref StatesQueue.vi"("error in (no error)"=w2373, "ref StatesQueue"=w2375, "State Machine in"=w2390) -> ("error out"=w2381:errorcluster, "State Machine out"=w2389:refnum<class "State Machine.lvclass">)  [unwired: 7 in]
            n1431 = disable-structure shown="Enabled" {
              disable-tunnel: [0 ("State") 45] -> w2397
              frame Enabled {
                # "Vai pra 0 para que\nos estados da fila \nsejam retirados."
              }
              frame Disabled {
                # "Verifica Texp\nantes de tudo."
              }
            }
            n1432 = call-dynamic "Write State.vi"("error in (no error)"=w2381, "State"=w2397, "State Machine in"=w2389) -> ("error out"=w2398:errorcluster, "State Machine out"=w2399:refnum<class "State Machine.lvclass">)  [unwired: 7 in]
            n1433 = call-dynamic "Write State Machine.vi"("error in (no error)"=w2398, "State Machine.lvclass"=w2399, "Device in"=w2400) -> ("error out"=w2395:errorcluster, "Device out"=w2396:refnum<class "Channel.lvclass">)  [unwired: 7 in]
          }
        }
        n1434 = call-dynamic "Write Channel.vi"("error in (no error)"=w2039, "Channel.lvclass"=w2040, "Acquisition in"=w2213) -> ("error out"=w2210:errorcluster, "Acquisition out"=w2209:refnum<class "Acquisition.lvclass">)  [unwired: 7 in]
        n1435 = call-dynamic "Write AcquisitionD.vi"("error in (no error)"=w2210, "Acquisition.lvclass"=w2209, "S4ACS_GUI in"=w2214) -> ("error out"=w2178:errorcluster, "S4ACS_GUI out"=w2182:refnum<class "S4GUI.lvclass">)  [unwired: 7 in]
        n1436 = Merge Errors(w2181, w2180, w2179, w2178) -> (w2177:errorcluster)
        n1437 = call "Write cfg file.vi"("error in (no error)"=w2177, "cfg file"="lastsaved.cfg", "S4ACS_GUI in"=w2182) -> ("error out"=w2264:errorcluster, "S4ACS_GUI out"=w2266:refnum<class "S4GUI.lvclass">)  [unwired: 7 in]
      }
      event "Frame Transfer", "AQM", "SZM", "EM Gain": Value Change {
        # "criar  S4GUI:CalcTemp.vi (metodo da classe S4GUI.lvclass)\na mesma lógica do Channel:ValidateConfig.vi usando\no cluster S4GUI:Parameters CCD em vez do cluster Interface:CCD CF.\nIgnore o Texp Min e apenas salve a temperatura em S4GUI:PrevTemp"
        # "Sinaliza que não há requisição de SET CCD mode"
        n1438 = event-data() -> ()  [unwired: 1 in, 6 out]
        n1439 = call-dynamic "Write SET request.vi"("error in (no error)"=w2458, "SET request"=FALSE, "S4GUI in"=w2460) -> ("error out"=w2457:errorcluster, "S4GUI out"=w2459:refnum<class "S4GUI.lvclass">)  [unwired: 7 in]
        n1440 = local read "Frame Transfer"() -> (w2473:enum16{"OFF", "ON"})
        n1441 = local read "EM Gain"() -> (w2462:u16)
        n1442 = local read "AQM"() -> (w2472:T4)
        n1443 = local read "SZM"() -> (w2471:T3)
        n1444 = call-dynamic "Read CCD mode.vi"("error in (no error)"=w2457, "S4GUI in"=w2459) -> ("error out"=w2470:errorcluster, "CCD mode"=w2475:T30, "S4GUI out"=w2476:refnum<class "S4GUI.lvclass">)  [unwired: 7 in]
        n1445 = Bundle By Name(cluster=w2475, "FTM"=w2473, "AQM"=w2472, "SZM"=w2471, "EM gain"=w2462) -> (w2474:T30)
        n1446 = call-dynamic "Write CCD mode.vi"("error in (no error)"=w2470, "CCD mode"=w2474, "S4GUI in"=w2476) -> ("error out"=w2468:errorcluster, "S4GUI out"=w2469:refnum<class "S4GUI.lvclass">)  [unwired: 7 in]
        n1447 = call-dynamic "LoadCCDmode.vi"("error in (no error)"=w2468, "S4GUI in"=w2469) -> ("error out"=w2466:errorcluster, "S4GUI out"=w2467:refnum<class "S4GUI.lvclass">)  [unwired: 8 in]
        n1448 = call-dynamic "Read Parameters CCD modes.vi"("error in (no error)"=w2466, "S4GUI in"=w2467) -> ("error out"=w2463:errorcluster, "Parameters CCD modes"=w2461:T5, "S4GUI out"=w2465:refnum<class "S4GUI.lvclass">)  [unwired: 7 in]
        n1449 = call-dynamic "Read InfoCCDmode.vi"("error in (no error)"=w2463, "S4GUI in"=w2465) -> ("error out"=w2453:errorcluster, "InfoCCDmode"=w2464:T2, "S4GUI out"=w2454:refnum<class "S4GUI.lvclass">)  [unwired: 7 in]
        n1450 = local write "Parameters CCD modes"(w2461) -> ()
        n1451 = local write "InfoCCDmode"(w2464) -> ()
        n1452 = call-dynamic "CalcTemp.vi"("error in (no error)"=w2453, "S4GUI in"=w2454) -> ("error out"=w2452:errorcluster, "S4GUI out"=w2451:refnum<class "S4GUI.lvclass">)  [unwired: 8 in]
        n1453 = call-dynamic "Read Prev Temp.vi"("error in (no error)"=w2452, "S4GUI in"=w2451) -> ("Prev Temp"=→"Preview Temp.":dbl)  [unwired: 7 in, 2 out]
      }
      event "TCS mode": Value Change {
        # "2024-04-04: Não se usa mais o ID para configurar a comunicação..."
        # "simul"
        # "real"
        # "Inicializar nova comunicação, de acordo\n com valor de TCS mode\n\nServer.Write id (T=6 ou F=12)\nTCS.Init"
        # "Parar a comunciação atual\nServer.End"
        n1454 = event-data() -> ("NewVal"=w2479:bool)  [unwired: 1 in, 5 out]
        n1455 = call-dynamic "Read TCS.lvclass.vi"("error in (no error)"=w2489, "S4GUI in"=w2490) -> ("error out"=w2484:errorcluster, "TCS.lvclass"=w2487:refnum<class "TCS.lvclass">, "S4GUI out"=w2488:refnum<class "S4GUI.lvclass">)  [unwired: 7 in]
        n1456 = call-dynamic "End.vi"("error in (no error)"=w2484, "Server in"=w2487) -> ("error out"=w2483:errorcluster, "Server out"=w2486:refnum<class "TCS.lvclass">)  [unwired: 8 in]
        n1457 = Select(t=u32 6, s=w2479, f=u32 12) -> (s? t:f=w2493:u32)
        n1458 = call-dynamic "Write id.vi"("error in (no error)"=w2483, "id"=w2493, "Server in"=w2486) -> ("error out"=w2482:errorcluster, "Server out"=w2485:refnum<class "TCS.lvclass">)  [unwired: 7 in]
        n1459 = call-dynamic "Initialize.vi"("error in (no error)"=w2482, "TCS in"=w2485) -> ("error out"=w2480:errorcluster, "TCS out"=w2481:refnum<class "TCS.lvclass">)  [unwired: 8 in]
        n1460 = call-dynamic "Write TCS.lvclass.vi"("error in (no error)"=w2480, "TCS.lvclass"=w2481, "S4GUI in"=w2488) -> ("error out"=w2477:errorcluster, "S4GUI out"=w2478:refnum<class "S4GUI.lvclass">)  [unwired: 7 in]
      }
      event "enter password": Value Change {
        n1461 = event-data() -> ("NewVal"=w2494:bool)  [unwired: 1 in]
        n1462 = case shown="True" w2494 {
          tunnel: [w2500 w2502] -> w2498
          tunnel: [w2499 w2501] -> w2497
          tunnel: w2496 -> [w2500 w2515]
          tunnel: w2495 -> [w2499 w2514]
          frame False {
          }
          frame True {
            # "Verifica senha de configuração de CCD do Administrador"
            n1463 = Equal?(x="password", y="camerasetup") -> (x = y?=w2512:bool)
            n1464 = call-dynamic "Write mode Adm.vi"("error in (no error)"=w2514, "mode Adm"=w2512, "S4GUI in"=w2515) -> ("error out"=w2503:errorcluster, "S4GUI out"=w2504:refnum<class "S4GUI.lvclass">)  [unwired: 7 in]
            n1465 = call-dynamic "Read mode Adm.vi"("error in (no error)"=w2503, "S4GUI in"=w2504) -> ("error out"=w2510:errorcluster, "mode Adm"=w2507:bool, "S4GUI out"=w2509:refnum<class "S4GUI.lvclass">)  [unwired: 7 in]
            n1466 = Select(t="Eng/Camera tab: password OK clicked successful" ("User Event"), s=w2507, f="Eng/Camera tab: password OK clicked with wrong input" ("User Event")) -> (s? t:f=w2508:string)
            n1467 = call-dynamic "Write User Event.vi"("error in (no error)"=w2510, "User Event"=w2508, "S4GUI in"=w2509) -> ("error out"=w2501:errorcluster, "S4GUI out"=w2502:refnum<class "S4GUI.lvclass">)  [unwired: 7 in]
          }
        }
      }
      event "enter password 2": Value Change {
        # "Verificação de senha na aba \"CCD modes\""
        n1468 = event-data() -> ("NewVal"=w2516:bool)  [unwired: 1 in]
        n1469 = case shown="True" w2516 {
          tunnel: [w2522 w2532] -> w2520
          tunnel: [w2521 w2531] -> w2519
          tunnel: w2518 -> [w2522 w2537]
          tunnel: w2517 -> [w2521 w2536]
          frame False {
          }
          frame True {
            # "Verifica senha de configuração de CCD do Administrador"
            n1470 = Equal?(x="password 2", y="ccdmodessetup") -> (x = y?=w2534:bool)
            n1471 = call-dynamic "Write mode Adm.vi"("error in (no error)"=w2536, "mode Adm"=w2534, "S4GUI in"=w2537) -> ("error out"=w2529:errorcluster, "S4GUI out"=w2530:refnum<class "S4GUI.lvclass">)  [unwired: 7 in]
            n1472 = call-dynamic "Read mode Adm.vi"("error in (no error)"=w2529, "S4GUI in"=w2530) -> ("error out"=w2527:errorcluster, "mode Adm"=w2524:bool, "S4GUI out"=w2528:refnum<class "S4GUI.lvclass">)  [unwired: 7 in]
            n1473 = Select(t="CCD mode tab: password OK clicked successful" ("User Event"), s=w2524, f="CCD mode tab: password OK clicked with wrong input" ("User Event")) -> (s? t:f=w2525:string)
            n1474 = call-dynamic "Write User Event.vi"("error in (no error)"=w2527, "User Event"=w2525, "S4GUI in"=w2528) -> ("error out"=w2531:errorcluster, "S4GUI out"=w2532:refnum<class "S4GUI.lvclass">)  [unwired: 7 in]
          }
        }
      }
      event "Tab ObsEng": Value Change {
        n1475 = event-data() -> ("NewVal"=w2538:enum32{"Obs", "CCD modes", "Guider", "Eng"})  [unwired: 1 in]
        n1476 = case shown="Default" w2538 {
          tunnel: [w2552 w2704 w2715] -> w2542
          tunnel: [w2554 w2702 w2713] -> w2541
          tunnel: w2540 -> [w2549 w2710 w2719]
          tunnel: w2539 -> [w2548 w2601 w2714]
          frame "CCD modes" {
            # "Sinaliza que não há requisição de SET CCD mode"
            # "Entrou na aba \"CCD modes\", ajusta para modo usuário normal..."
            n1477 = call-dynamic "Read TabAcqType index.vi"("error in (no error)"=w2548, "S4GUI in"=w2549) -> ("error out"=w2547:errorcluster, "TabAcqType index"=w2545:u32, "S4GUI out"=w2546:refnum<class "S4GUI.lvclass">)  [unwired: 7 in]
            n1478 = case shown="4" w2545 {
              tunnel: w2547 -> [w2584 w2589]
              tunnel: [w2583 w2588] -> w2550
              tunnel: [w2582 w2587] -> w2544
              tunnel: [FALSE ("Visible") TRUE ("Visible")] -> w2543
              frame 0, Default {
                n1479 = local read "Frame Transfer"() -> (w2582:enum16{"OFF", "ON"})
                n1480 = property on="Frame Transfer" class="Enum (strict)"(error in=w2584, "DisabledEnum"=T12."Enabled" ("Disabled")) -> (error out=w2583:errorcluster)  [unwired: 1 in, 1 out]
              }
              frame 4 {
